vi "getHWIO_3_statusBusy.vi"(0 "Camera in":refnum<class "Camera.lvclass">, 5 "error in (no error)":errorcluster) -> (14 "Camera out":refnum<class "Camera.lvclass">, 15 "on":bool=TRUE, 16 "polarity":u16(ring)=1 items=["high level"=1, "low level"=2], 17 "signal_type":u32(ring) items=["Status Busy", "Status Expos", "Status Line", "Status Armed"], 19 "error out":errorcluster)   [LabVIEW 2019, in "Camera.lvclass"]
doc: "Gets polarity, status (enabled / disabled), and also fuction (exposure or line) of HWIO 3 status busy. Generates an error if camera is recording or if HWIO configuration is not supported."
uses:
  Camera.lvclass
  pco.sdk/TimingControl/TimingControl.lvlib
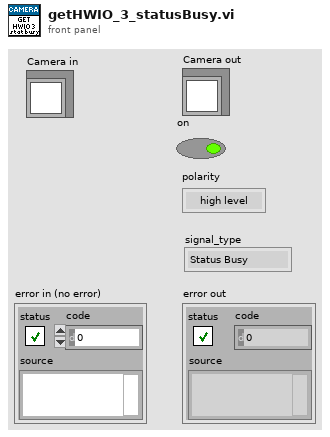
[diagram p1: front panel]
types:
  T1 = cluster{"wSignalNum":u16, "wEnabled":u16, "wType":u16, "wPolarity":u16, "wFilterSetting":u16, "wSelected":u16, "dwParameter":u32[], "dwSignalFunctionality":u32[]}
  T2 = cluster{"strSignalName":string[], "wSignalDefinitions":u16, "wSignalTypes":u16, "wSignalPolarity":u16, "wSignalFilter":u16}
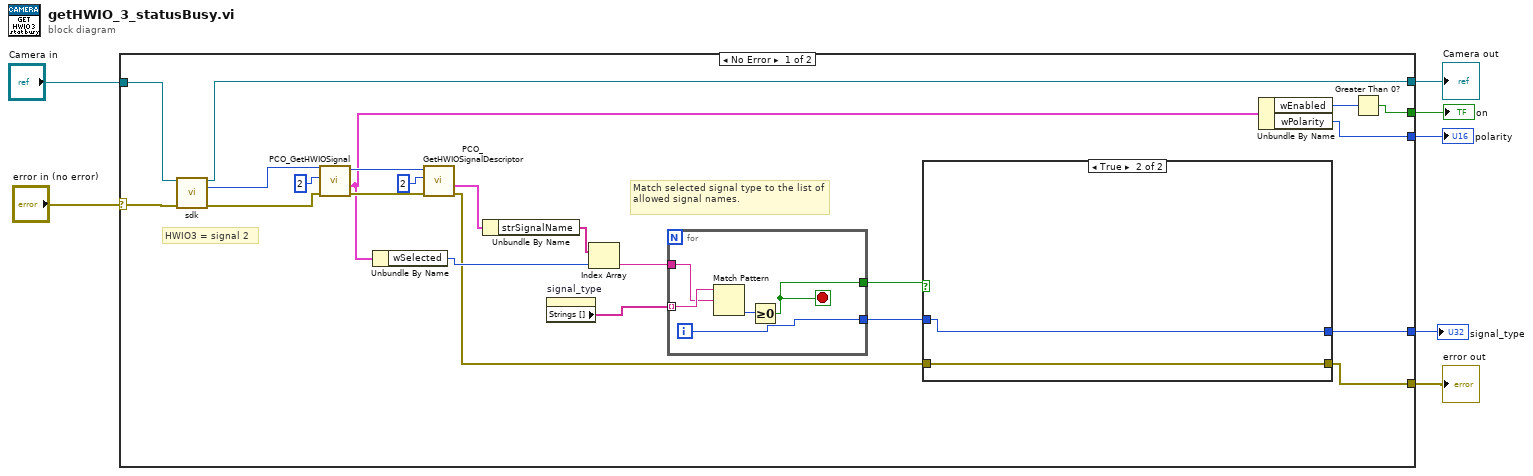
[diagram p0: block diagram]
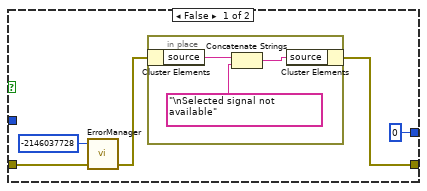
[diagram p2: hidden frame]
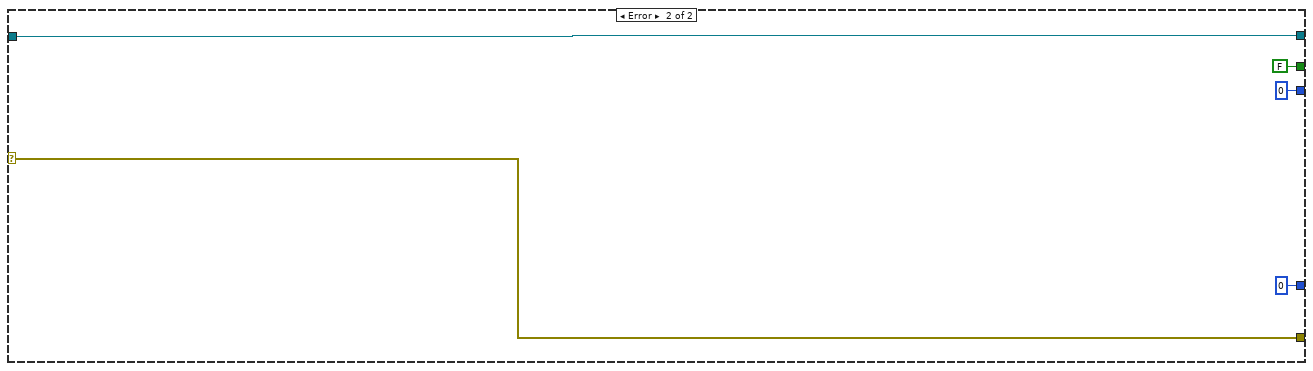
[diagram p3: hidden frame]
diagram:
  n1 = case shown="No Error" "error in (no error)" {
    selector: "error in (no error)" -> [w29 w50]
    tunnel: [w14 w50] -> w6
    tunnel: "Camera in" -> [w30 w49]
    tunnel: [w9 w49] -> w4
    tunnel: [w13 0] -> w3
    tunnel: [w11 FALSE] -> w2
    tunnel: [w10 u16 0 ("wPolarity")] -> w1
    frame No Error {
      # "Match selected signal type to the list of allowed signal names."
      # "HWIO3 = signal 2"
      n2 = call-dynamic "sdk.vi"("Camera in"=w30, "error in (no error)"=w29) -> ("Camera out"=w9:refnum<class "Camera.lvclass">, "sdk"=w20:u64, "error out"=w19:errorcluster)  [unwired: 11 in]
      n3 = call "PCO_GetHWIOSignal.vi"("error in (no error)"=w19, "wSignalNum"=u16 2, "ph"=w20) -> ("error out"=w27:errorcluster, "strSignal"=w18:T1, "ph out"=w26:u64)  [unwired: 5 in, 1 out]
      n4 = Unbundle By Name(w18) -> ("wSelected"=w17:u16)
      n5 = call "PCO_GetHWIOSignalDescriptor.vi"("error in (no error)"=w27, "wSignalNum"=u16 2, "ph"=w26) -> ("error out"=w8:errorcluster, "strSignalDesc"=w24:T2)  [unwired: 5 in, 2 out]
      n6 = Unbundle By Name(w24) -> ("strSignalName"=w16:string[])
      n7 = property on="signal_type" class="Ring (strict)"() -> ("Strings []"=w23:string[])  [unwired: 2 in, 2 out]
      n8 = Index Array(array=w16, index=w17) -> (element=w15:string)
      n9 = for {
        tunnel: [w44] -> w21
        tunnel: [w43] -> w22
        tunnel: w23 -> [w42] mode=indexing
        tunnel: w15 -> [w41]
        i -> [w44]
        stop <- w43 stop-if-true
        n10 = Match Pattern(string=w42, regular expression=w41) -> (offset past match=w45:i32)  [unwired: 1 in, 3 out]
        n11 = Greater Or Equal To 0?(x=w45) -> (x >= 0?=w43:bool)
      }
      n12 = case shown="True" w22 {
        tunnel: w8 -> [w35 w40]
        tunnel: [w32 w40] -> w14
        tunnel: w21 -> [_ w39]
        tunnel: [0 w39] -> w13
        frame False {
          n13 = call "ErrorManager.vi"("error in (no error)"=w35, "error code"=-2146037728) -> ("error out"=w33:errorcluster)  [unwired: 2 in, 1 out]
          n14 = in-place {
            n15 = in-place-cluster #1(w33) -> ("source"=w38:string)
            n16 = Concatenate Strings(w38, "\nSelected signal not available" ("string")) -> (w37:string)
            n17 = in-place-cluster #1("source"=w37) -> (w32:errorcluster)
          }
        }
        frame True {
        }
      }
      n18 = Unbundle By Name(w18) -> ("wEnabled"=w12:u16, "wPolarity"=w10:u16)
      n19 = Greater Than 0?(x=w12) -> (x > 0?=w11:bool)
    }
    frame Error {
    }
  }
  "Camera out" <- w4
  "error out" <- w6
  "signal_type" <- w3
  "on" <- w2
  "polarity" <- w1
